vi "Test My Cloneable Module API.vi"() -> ()   [LabVIEW 2023]
doc: "My Module API Tester.\n_____\nBased on DQMH Project Template 6.1.0.94."
uses:
  <vilib>/Utility/error.llb/DialogType.ctl
  My Cloneable Module.lvlib
panel:
  in  "Show Diagram on Init":bool
  in  "wait for reply":bool=TRUE
  in  "Run as Singleton?":bool
  in  "Show Block Diagram":bool
  in  "Refresh Modules":bool
  in  "X":dbl=1.0
  out "Reply Payload":dbl
  out "Active Modules":string[](array[string])
  in  "Stop Module":bool
  in  "Select Module":i32(ring)=-1 caption="Select Module\nTo send Request to" items=["All"=-1]
  in  "Run New Module":bool
  out "Do Something Count":i32
  in  "Test Do Something Else and Wait for Reply":bool
  in  "Hide Module Panel":bool
  in  "Show Module Panel":bool
  in  "Test Do Something Else":bool
  in  "Test Do Something":bool
  out "Status":string
  # "This VI tests the API for the Module."
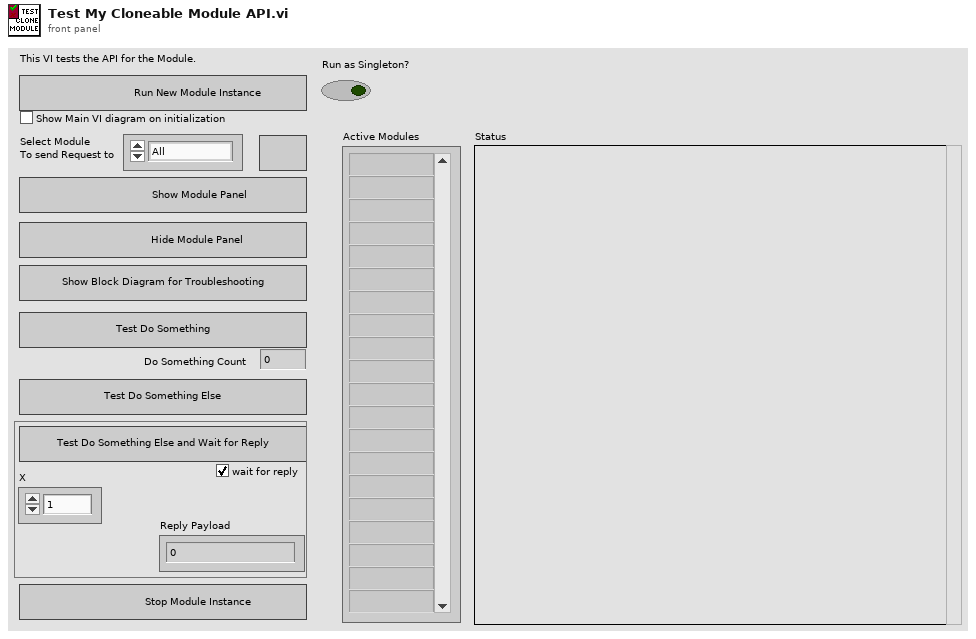
[diagram p1: front panel]
types:
  T1 = typedef "My Cloneable Module.lvlib/Broadcast Events--cluster.ctl" = cluster{"Module Did Init":refnum<user-event>, "Status Updated":refnum<user-event>, "Error Reported":refnum<user-event>, "Did Something":refnum<user-event>, "Module Did Stop":refnum<user-event>, "Update Module Execution Status":refnum<user-event>}
  T2 = typedef "DialogType.ctl" = u16
  T3 = typedef "My Cloneable Module.lvlib/Do Something Else and Wait (Reply Payload)--cluster.ctl" = cluster{"Value":dbl, "error":errorcluster}
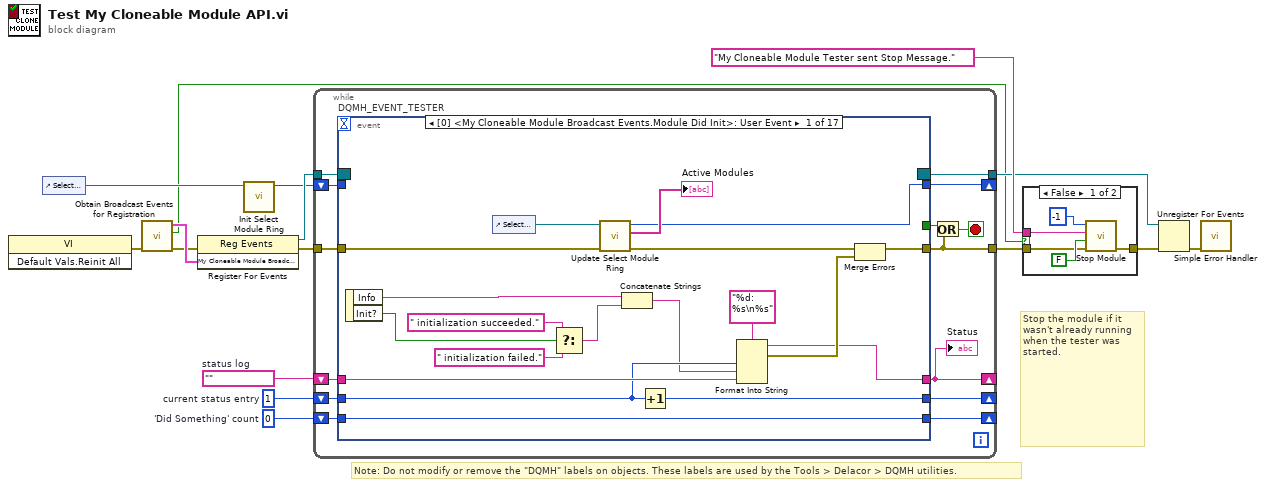
[diagram p0: block diagram]
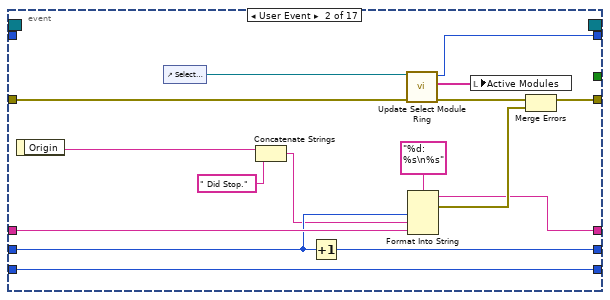
[diagram p3: hidden frame]
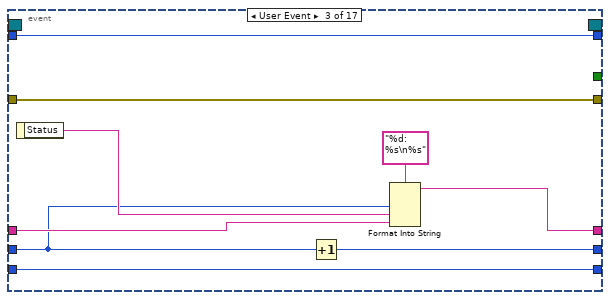
[diagram p4: hidden frame]
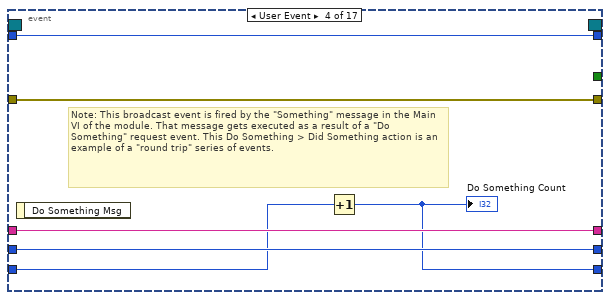
[diagram p5: hidden frame]
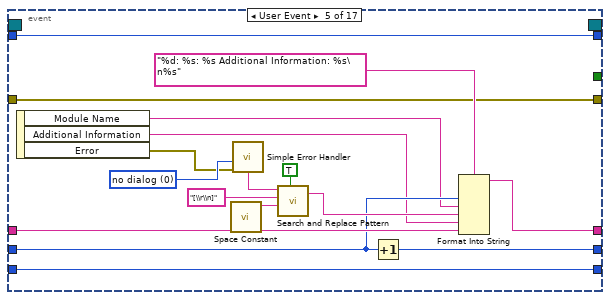
[diagram p6: hidden frame]
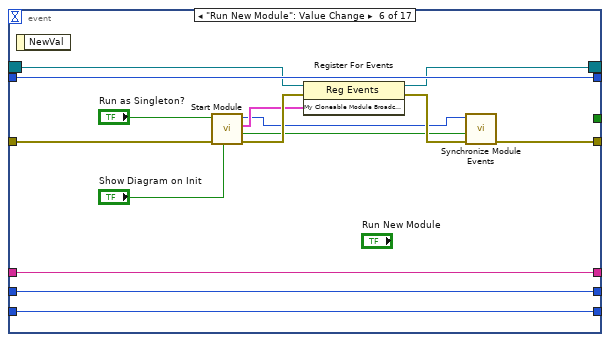
[diagram p7: hidden frame]
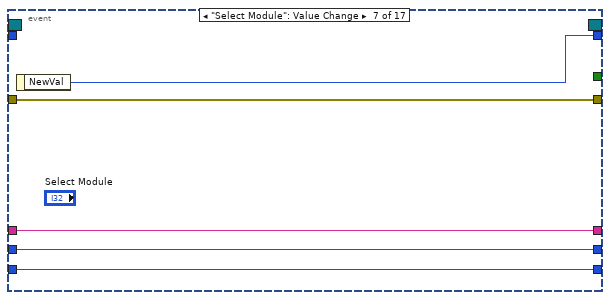
[diagram p8: hidden frame]
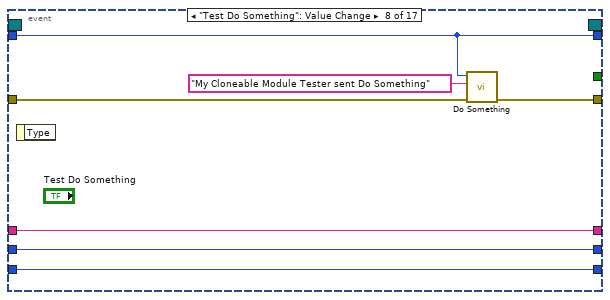
[diagram p9: hidden frame]
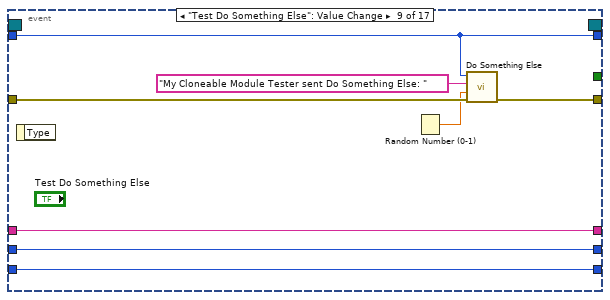
[diagram p10: hidden frame]
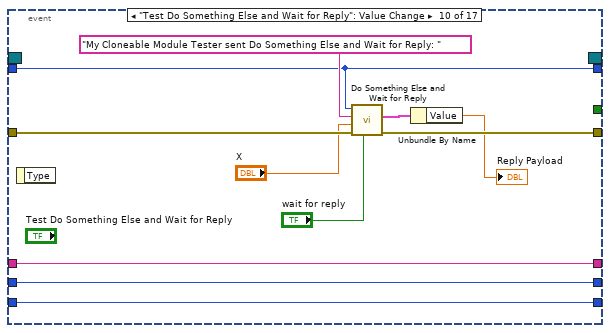
[diagram p11: hidden frame]
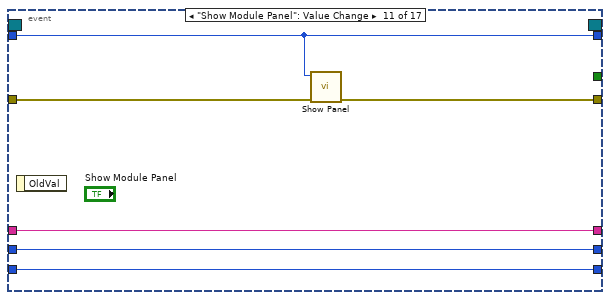
[diagram p12: hidden frame]
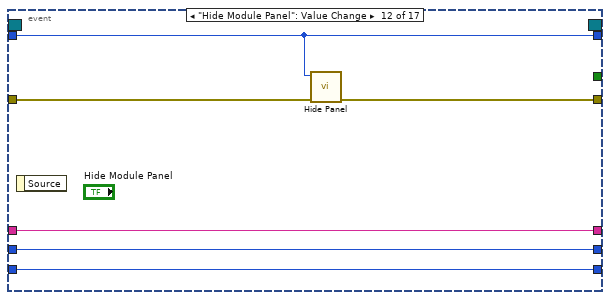
[diagram p13: hidden frame]
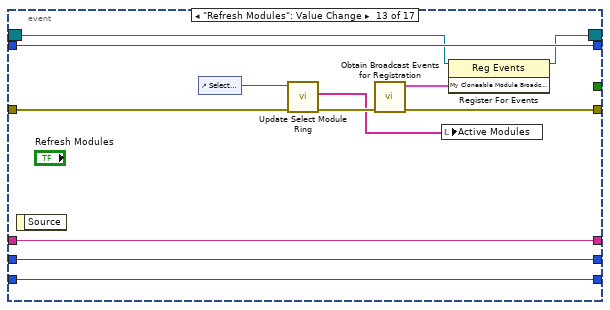
[diagram p14: hidden frame]
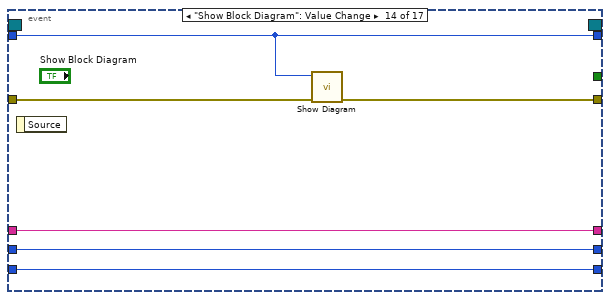
[diagram p15: hidden frame]
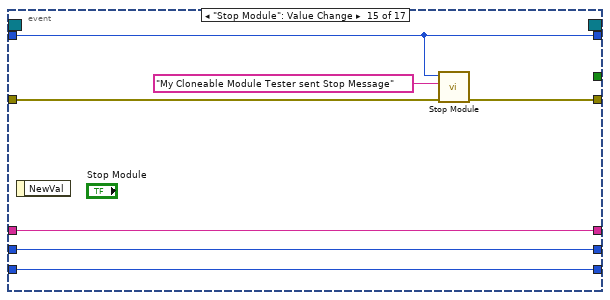
[diagram p16: hidden frame]
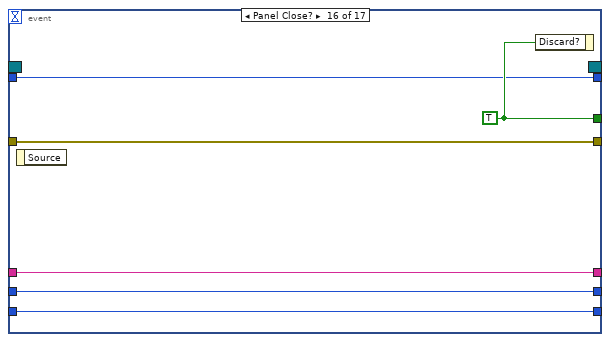
[diagram p17: hidden frame]
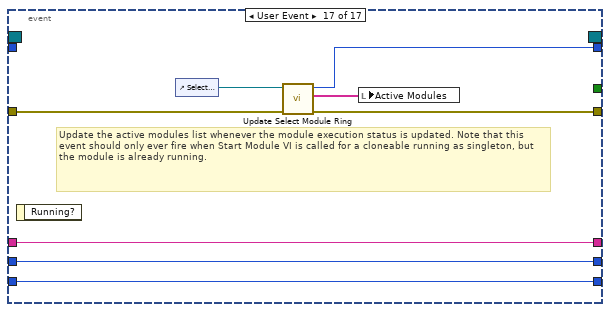
[diagram p18: hidden frame]
diagram:
  w12 = 0  # 'Did Something' count
  w13 = 1  # current status entry
  w14 = ""  # status log
  # "Stop the module if it wasn't already running when the tester was started."
  # "Note: Do not modify or remove the \"DQMH\" labels on objects. These labels are used by the Tools > Delacor > DQMH utilities."
  n1 = invoke class="VI" method="Default Vals.Reinit All"() -> (error out=w5:errorcluster)  [unwired: 3 in, 2 out]
  n2 = control-ref of="Select Module"() -> (w10:refnum<vi>)
  n3 = call "Obtain Broadcast Events for Registration.vi"("error in"=w5) -> ("error out"=w4:errorcluster, "Already running?"=w3:bool, "My Cloneable Module Broadcast Events"=w9:T1)  [unwired: 8 in]
  n4 = register-events(error in=w4, w9) -> (reference out=w16:refnum<event-registration>, error out=w8:errorcluster)  [unwired: 1 in]
  n5 = call "Init Select Module Ring.vi"("Select Module Ring Ref"=w10) -> ("Value for All Modules"=w11:i32)  [unwired: 8 in, 2 out]
  n6 = while {
    tunnel: w16 -> [w30]
    tunnel: [w17] -> w2
    tunnel: w8 -> [w28]
    shift-right: [w24] -> _
    shift-left: w14 -> [w26]
    shift-right: [w25] -> _
    shift-left: w13 -> [w27]
    shift-right: [w22] -> _
    shift-left: w12 -> [w23]
    shift-right: [w19] -> _
    shift-left: w11 -> [w20]
    tunnel: [w18] -> w6
    stop <- w21 stop-if-true
    n7 = event "DQMH_EVENT_TESTER" shown="[0] <My Cloneable Module Broadcast Events.Module Did Init>: User Event" {
      selector: w30 -> [_ _ _ _ _ w105 _ _ _ _ _ _ w161 _ _ _ _]
      dyn-events: [_ _ _ _ _ w104 _ _ _ _ _ _ w160 _ _ _ _] -> w18
      timeout: _ -> [_ _ _ _ _ _ _ _ _ _ _ _ _ _ _ _ _]
      tunnel: [_ _ _ _ _ _ _ _ _ _ _ _ _ _ _ w186 _] -> w29
      tunnel: [w38 w56 w74 w80 w84 w103 w117 w123 w131 w143 w148 w154 w157 w169 w175 w185 w189] -> w17
      tunnel: w28 -> [w40 w58 w74 w80 w84 w106 w117 w124 w132 w135 w149 w155 w162 w173 w176 w185 w190]
      tunnel: w27 -> [w46 w62 w66 w78 w87 w109 w115 w120 w127 w140 w146 w152 w166 w171 w179 w183 w193]
      tunnel: w26 -> [w47 w63 w70 w79 w88 w110 w116 w121 w128 w141 w147 w153 w167 w172 w180 w184 w194]
      tunnel: [w44 w60 w71 w79 w86 w110 w116 w121 w128 w141 w147 w153 w167 w172 w180 w184 w194] -> w24
      tunnel: [w45 w61 w73 w78 w85 w109 w115 w120 w127 w140 w146 w152 w166 w171 w179 w183 w193] -> w25
      tunnel: w23 -> [w41 w59 w69 w77 w97 w108 w114 w119 w126 w139 w145 w151 w165 w170 w178 w182 w192]
      tunnel: [w41 w59 w69 w76 w97 w108 w114 w119 w126 w139 w145 w151 w165 w170 w178 w182 w192] -> w22
      tunnel: w20 -> [_ _ w67 w75 w96 w107 _ w118 w125 w138 w144 w150 w164 w168 w177 w181 _]
      tunnel: [w35 w53 w67 w75 w96 w107 w113 w118 w125 w138 w144 w150 w164 w168 w177 w181 w188] -> w19
      event User Event {
        n8 = event-data() -> ("Info"=w43:string, "Init?"=w32:bool)  [unwired: 1 in]
        n9 = control-ref of="Select Module"() -> (w37:refnum<vi>)
        n10 = Select(t=" initialization succeeded.", s=w32, f=" initialization failed.") -> (s? t:f=w31:string)
        n11 = call "Update Select Module Ring.vi"("error in (no error)"=w40, "Select Module Ring Ref"=w37) -> ("error out"=w39:errorcluster, "Active Modules (Array)"=→"Active Modules":string[], "New Module Ring Value"=w35:i32)  [unwired: 7 in]
        n12 = Concatenate Strings(w43, w31) -> (w42:string)
        n13 = Increment(x=w46) -> (x+1=w45:i32)
        n14 = Format Into String(format string="%d: %s\n%s", w46, w42, w47) -> (resulting string=w44:string, error out=w49:errorcluster)  [unwired: 2 in]
        n15 = Merge Errors(w39, w49) -> (w38:errorcluster)
      }
      event User Event {
        n16 = event-data() -> ("Origin"=w51:string)  [unwired: 1 in]
        n17 = control-ref of="Select Module"() -> (w55:refnum<vi>)
        n18 = Concatenate Strings(w51, " Did Stop.") -> (w50:string)
        n19 = Increment(x=w62) -> (x+1=w61:i32)
        n20 = call "Update Select Module Ring.vi"("error in (no error)"=w58, "Select Module Ring Ref"=w55) -> ("error out"=w57:errorcluster, "Active Modules (Array)"=w54:string[], "New Module Ring Value"=w53:i32)  [unwired: 7 in]
        n21 = Format Into String(format string="%d: %s\n%s", w62, w50, w63) -> (resulting string=w60:string, error out=w65:errorcluster)  [unwired: 2 in]
        n22 = local write "Active Modules"(w54) -> ()
        n23 = Merge Errors(w57, w65) -> (w56:errorcluster)
      }
      event User Event {
        n24 = event-data() -> ("Status"=w68:string)  [unwired: 1 in]
        n25 = Increment(x=w66) -> (x+1=w73:i32)
        n26 = Format Into String(format string="%d: %s\n%s", w66, w68, w70) -> (resulting string=w71:string)  [unwired: 2 in, 1 out]
      }
      event User Event {
        # "Note: This broadcast event is fired by the \"Something\" message in the Main VI of the module. That message gets executed as a result of a \"Do Something\" request event. This Do Something > Did Something action is an example of a \"round trip\" series of events."
        n27 = event-data() -> ()  [unwired: 1 in, 1 out]
        n28 = Increment(x=w77) -> (x+1=w76:i32)
        "Do Something Count" <- w76
      }
      event User Event {
        w89 = T2 0 items=["no dialog", "OK message", "continue or stop message", "OK message + warnings", "continue/stop + warnings"] ("type of dialog (OK msg:1)")
        n29 = event-data() -> ("Module Name"=w83:string, "Additional Information"=w82:string, "Error"=w81:errorcluster)  [unwired: 1 in]
        n30 = call <vilib>:"Space Constant.vi"() -> ("String"=w93:string)
        n31 = call <vilib>:"Simple Error Handler.vi"("type of dialog (OK msg:1)"=w89, "error in (no error)"=w81) -> ("message"=w90:string)  [unwired: 3 in, 4 out]
        n32 = call <vilib>:"Search and Replace Pattern.vi"("string"=w90, "regular expression (\"\")"="[\\r\\n]" ("regular expression (\"\")"), "replace string (\"\")"=w93, "replace all? (F)"=TRUE ("replace all CR/LF with spaces")) -> ("result string"=w91:string)  [unwired: 1 in, 1 out]
        n33 = Increment(x=w87) -> (x+1=w85:i32)
        n34 = Format Into String(format string="%d: %s: %s Additional Information: %s\n%s", w87, w83, w91, w82, w88) -> (resulting string=w86:string)  [unwired: 2 in, 1 out]
      }
      event "Run New Module": Value Change {
        n35 = event-data() -> ()  [unwired: 1 in, 1 out]
        n36 = call "Start Module.vi"("Show Main VI Diagram on Init (F)"="Show Diagram on Init", "error in"=w106, "Run as Singleton? (F)"="Run as Singleton?") -> ("error out"=w111:errorcluster, "Wait for Event Sync?"=w102:bool, "My Cloneable Module Broadcast Events"=w101:T1, "Module ID"=w98:i32)  [unwired: 5 in]
        n37 = register-events(reference=w105, error in=w111, w101) -> (reference out=w104:refnum<event-registration>, error out=w112:errorcluster)
        n38 = call "Synchronize Module Events.vi"("error in"=w112, "Wait for Event Sync?"=w102, "Module ID in"=w98) -> ("error out"=w103:errorcluster)  [unwired: 7 in, 1 out]
      }
      event "Select Module": Value Change {
        n39 = event-data() -> ("NewVal"=w113:i32)  [unwired: 1 in]
      }
      event "Test Do Something": Value Change {
        n40 = event-data() -> ()  [unwired: 1 in, 1 out]
        n41 = call "Do Something.vi"("error in (no error)"=w124, "Do Something Message"="My Cloneable Module Tester sent Do Something", "Module ID"=w118) -> ("error out"=w123:errorcluster)  [unwired: 8 in]
      }
      event "Test Do Something Else": Value Change {
        n42 = event-data() -> ()  [unwired: 1 in, 1 out]
        n43 = Random Number (0-1)() -> (number: 0 to 1=w129:dbl)
        n44 = call "Do Something Else.vi"("error in (no error)"=w132, "X"=w129, "Do Something else Message"="My Cloneable Module Tester sent Do Something Else: " ("Do Something Message"), "Module ID"=w125) -> ("error out"=w131:errorcluster)  [unwired: 7 in]
      }
      event "Test Do Something Else and Wait for Reply": Value Change {
        n45 = event-data() -> ()  [unwired: 1 in, 1 out]
        n46 = call "Do Something Else and Wait for Reply.vi"("wait for reply (T)"="wait for reply", "error in (no error)"=w135, "X"="X", "Do Something Else Message"="My Cloneable Module Tester sent Do Something Else and Wait for Reply: " ("Do Something Message"), "Module ID"=w138) -> ("error out"=w143:errorcluster, "Reply Payload"=w137:T3)  [unwired: 4 in, 1 out]
        n47 = Unbundle By Name(w137) -> ("Value"=→"Reply Payload":dbl)
      }
      event "Show Module Panel": Value Change {
        n48 = event-data() -> ()  [unwired: 1 in, 1 out]
        n49 = call "Show Panel.vi"("error in (no error)"=w149, "Module ID"=w144) -> ("error out"=w148:errorcluster)  [unwired: 9 in]
      }
      event "Hide Module Panel": Value Change {
        n50 = event-data() -> ()  [unwired: 1 in, 1 out]
        n51 = call "Hide Panel.vi"("error in (no error)"=w155, "Module ID"=w150) -> ("error out"=w154:errorcluster)  [unwired: 9 in]
      }
      event "Refresh Modules": Value Change {
        n52 = event-data() -> ()  [unwired: 1 in, 1 out]
        n53 = control-ref of="Select Module"() -> (w163:refnum<vi>)
        n54 = call "Update Select Module Ring.vi"("error in (no error)"=w162, "Select Module Ring Ref"=w163) -> ("error out"=w158:errorcluster, "Active Modules (Array)"=w156:string[])  [unwired: 7 in, 1 out]
        n55 = call "Obtain Broadcast Events for Registration.vi"("error in"=w158) -> ("error out"=w157:errorcluster, "My Cloneable Module Broadcast Events"=w159:T1)  [unwired: 8 in, 1 out]
        n56 = local write "Active Modules"(w156) -> ()
        n57 = register-events(reference=w161, w159) -> (reference out=w160:refnum<event-registration>)  [unwired: 1 in, 1 out]
      }
      event "Show Block Diagram": Value Change {
        n58 = event-data() -> ()  [unwired: 1 in, 1 out]
        n59 = call "Show Diagram.vi"("error in (no error)"=w173, "Module ID"=w168) -> ("error out"=w169:errorcluster)  [unwired: 9 in]
      }
      event "Stop Module": Value Change {
        n60 = event-data() -> ()  [unwired: 1 in, 1 out]
        n61 = call "Stop Module.vi"("error in"=w176, "Origin"="My Cloneable Module Tester sent Stop Message", "Module ID"=w177) -> ("error out"=w175:errorcluster)  [unwired: 8 in]
      }
      event Panel Close? {
        w186 = TRUE ("Discard?")
        n62 = event-data() -> ()  [unwired: 1 in, 1 out]
        n63 = event-data("Discard?"=w186) -> ()  [unwired: 1 in, 1 out]
      }
      event User Event {
        # "Update the active modules list whenever the module execution status is updated. Note that this event should only ever fire when Start Module VI is called for a cloneable running as singleton, but the module is already running."
        n64 = event-data() -> ()  [unwired: 1 in, 1 out]
        n65 = control-ref of="Select Module"() -> (w191:refnum<vi>)
        n66 = call "Update Select Module Ring.vi"("error in (no error)"=w190, "Select Module Ring Ref"=w191) -> ("error out"=w189:errorcluster, "Active Modules (Array)"=w187:string[], "New Module Ring Value"=w188:i32)  [unwired: 7 in]
        n67 = local write "Active Modules"(w187) -> ()
      }
    }
    "Status" <- w24
    n68 = Or(x=w29, y=w17) -> (x .or. y?=w21:bool)
  }
  n69 = case shown="False" w3 {
    tunnel: [w199 w200] -> w15
    tunnel: "My Cloneable Module Tester sent Stop Message." ("Origin") -> [w198 _]
    tunnel: w2 -> [w195 w200]
    frame False {
      n70 = call "Stop Module.vi"("error in"=w195, "Wait for Module to stop? (F)"=FALSE ("Wait for Module to stop?"), "Origin"=w198, "Module ID"=-1 ("Stop all")) -> ("error out"=w199:errorcluster)  [unwired: 7 in]
    }
    frame True {
    }
  }
  n71 = Unregister For Events(event registration refnum=w6, error in=w15) -> (error out=w1:errorcluster)
  n72 = call <vilib>:"Simple Error Handler.vi"("error in (no error)"=w1) -> ()  [unwired: 4 in, 5 out]
